vi "Format Endpoint Name.vi"(10 "Endpoint":string, 11 "Module Path":string) -> (2 "Formatted Endpoint Name":string, 3 "Full Endpoint Name":string)   [LabVIEW 2020, in "Routing and Faulting System Explorer.lvlib"]
uses:
  Routing and Faulting System Explorer.lvlib
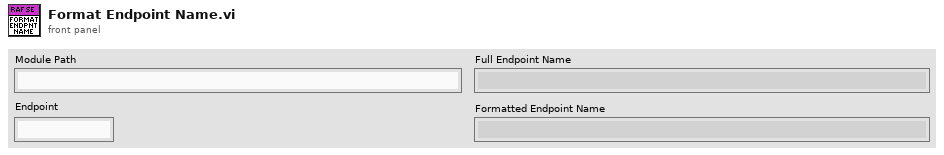
[diagram p1: front panel]
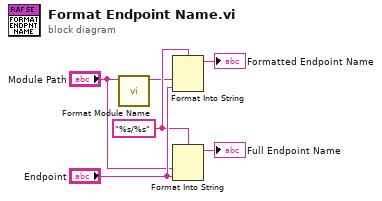
[diagram p0: block diagram]
diagram:
  w4 = "%s/%s" ("format string")
  n1 = call "Format Module Name.vi"("Module Path"="Module Path") -> ("Formatted Module Path"=w2:string)  [unwired: 10 in]
  n2 = Format Into String(format string=w4, w2, "Endpoint") -> (resulting string=→"Formatted Endpoint Name":string)  [unwired: 2 in, 1 out]
  n3 = Format Into String(format string=w4, "Module Path", "Endpoint") -> (resulting string=→"Full Endpoint Name":string)  [unwired: 2 in, 1 out]
